vi "onIncomingMessagingError.vi"(8 "error in (no error)":errorcluster, 10 "model in":refnum<class "IModel.lvclass">, 11 "State in":refnum<class "State.lvclass">) -> (0 "error out":errorcluster, 2 "model out":refnum<class "IModel.lvclass">, 3 "State out":refnum<class "State.lvclass">)   [LabVIEW 2012, in "State.lvclass"]
uses:
  State.lvclass
  IModel/IModel.lvclass
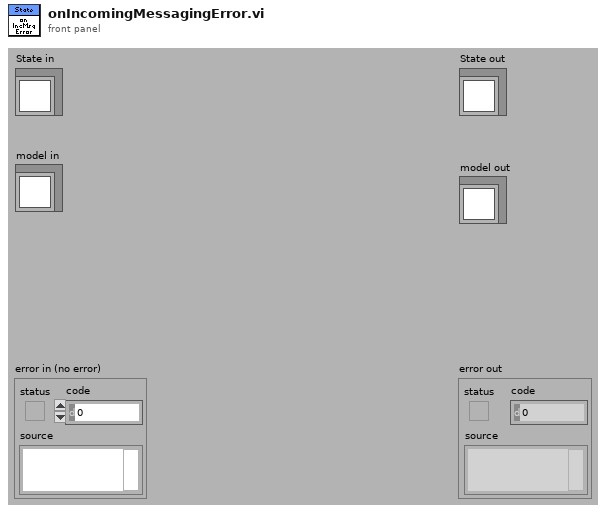
[diagram p1: front panel]
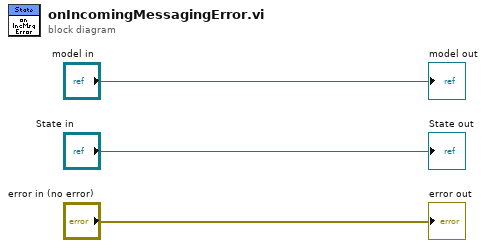
[diagram p0: block diagram]
diagram:
  "error out" <- "error in (no error)"
  "State out" <- "State in"
  "model out" <- "model in"
